vi "lidar_imitator.vi"(11 "error in (no error)":errorcluster) -> (2 "error out":errorcluster, 3 "array":dbl[][](array[numeric]))   [LabVIEW 2014]
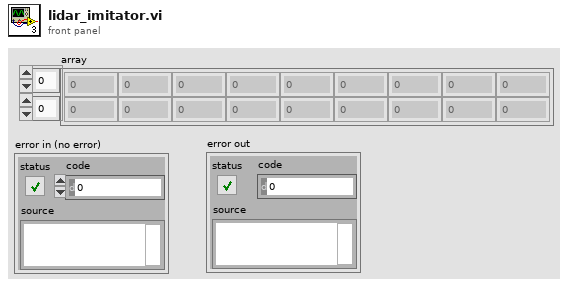
[diagram p1: front panel]
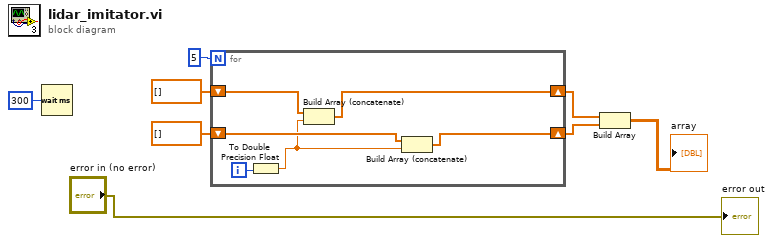
[diagram p0: block diagram]
diagram:
  n1 = Wait (ms)(milliseconds to wait=u32 300) -> ()  [unwired: 1 out]
  n2 = for {
    N: 5 -> [_]
    shift-right: [w13] -> w5
    shift-left: dbl[] [] -> [w14]
    shift-right: [w12] -> w4
    shift-left: dbl[] [] -> [w11]
    i -> [w10]
    n3 = To Double Precision Float(number=w10) -> (double precision float=w9:dbl)
    n4 = Build Array (concatenate)(w14, w9) -> (w13:dbl[])
    n5 = Build Array (concatenate)(w11, w9) -> (w12:dbl[])
  }
  n6 = Build Array(w5, w4) -> (→"array":dbl[][])
  "error out" <- "error in (no error)"
